vi "Get Byte Order.vi"(0 "VISA resource name":refnum<visa-resource-name>, 11 "error in (no error)":errorcluster) -> (4 "VISA resource name out":refnum<visa-resource-name>, 6 "Byte Order":string, 15 "error out":errorcluster)   [LabVIEW 2018, in "Keithley 2450.lvlib"]
doc: "This gets the byte order for the IEEE-754 binary formats."
uses:
  <instrlib>/Keithley 2450/Keithley 2450.lvlib
panel:
  out "Status":sgl[](array[numeric])
  out "Timestamp":sgl[](array[numeric])
  out "Resistance":sgl[](array[numeric])
  out "Current":sgl[](array[numeric])
  out "Voltage":sgl[](array[numeric])
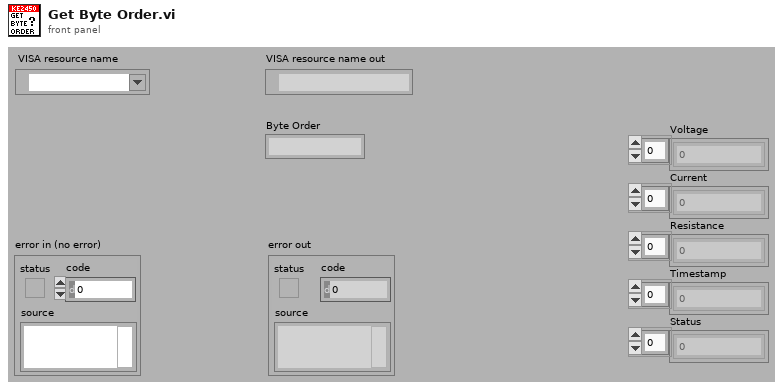
[diagram p1: front panel]
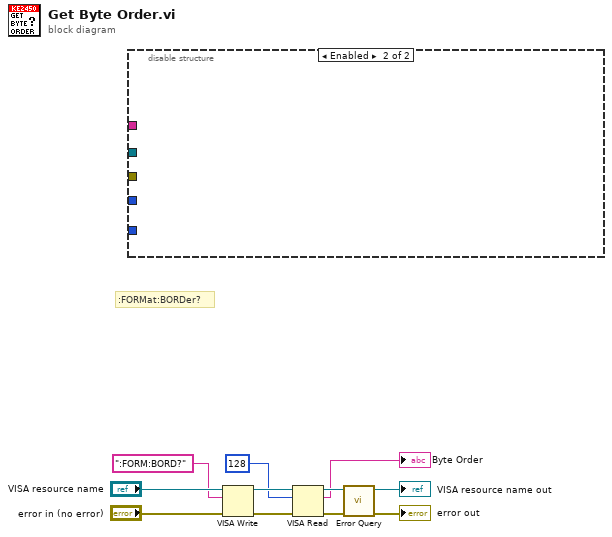
[diagram p0: block diagram]
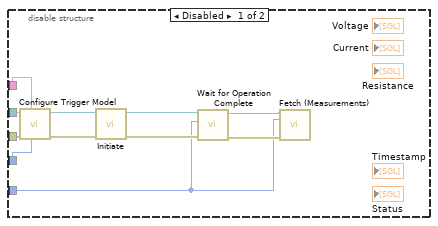
[diagram p2: hidden frame]
diagram:
  # ":FORMat:BORDer?"
  n1 = disable-structure shown="Enabled" {
    disable-tunnel: _ -> [w18 _]
    disable-tunnel: _ -> [w17 _]
    disable-tunnel: _ -> [w16 _]
    disable-tunnel: _ -> [w15 _]
    disable-tunnel: _ -> [w12 _]
    frame Disabled {
      n2 = call <instrlib>:"Configure Trigger Model.vi"("Trigger Count (1)"=w17, "Buffer Name (defbuffer1)"=w12, "error in (no error)"=w15, "VISA resource name"=w16) -> ("error out"=w13:errorcluster, "VISA resource name out"=w14:refnum<visa-resource-name>)  [unwired: 6 in]
      n3 = call <instrlib>:"Initiate.vi"("error in (no error)"=w13, "VISA resource name"=w14) -> ("error out"=w21:errorcluster, "VISA resource name out"=w22:refnum<visa-resource-name>)  [unwired: 8 out]
      n4 = call <instrlib>:"Wait for Operation Complete.vi"("error in (no error)"=w21, "Timeout (10000 ms)"=w18, "VISA resource name"=w22) -> ("error out"=w20:errorcluster, "VISA resource name out"=w19:refnum<visa-resource-name>)  [unwired: 7 out]
      n5 = call <instrlib>:"Fetch (Measurements).vi"("VISA resource name"=w19, "Timeout (10000 ms)"=w18, "error in (no error)"=w20) -> ()  [unwired: 2 in, 11 out]
    }
    frame Enabled {
    }
  }
  n6 = VISA Write(VISA resource name="VISA resource name", write buffer=":FORM:BORD?" ("Fetch Measurement"), error in (no error)="error in (no error)") -> (VISA resource name out=w7:refnum<visa-resource-name>, error out=w5:errorcluster)  [unwired: 1 out]
  n7 = VISA Read(VISA resource name=w7, byte count=u32 128, error in (no error)=w5) -> (VISA resource name out=w6:refnum<visa-resource-name>, read buffer=→"Byte Order":string, error out=w4:errorcluster)  [unwired: 1 out]
  n8 = call <instrlib>:"Error Query.vi"("error in (no error)"=w4, "VISA resource name"=w6) -> ("error out"=→"error out":errorcluster, "VISA resource name out"=→"VISA resource name out":refnum<visa-resource-name>)  [unwired: 8 out]
